vi "tearDown.vi"(8 "error in (no error)":errorcluster, 11 "LUnit test In":refnum<class "LUnit test 2.lvclass">) -> (0 "error out":errorcluster, 3 "LUnit test Out":refnum<class "LUnit test 2.lvclass">)   [LabVIEW 2020, in "LUnit test 2.lvclass"]
uses:
  LUnit test 2.lvclass
  <vilib>/Asteme/LUnit/Test Case.lvclass
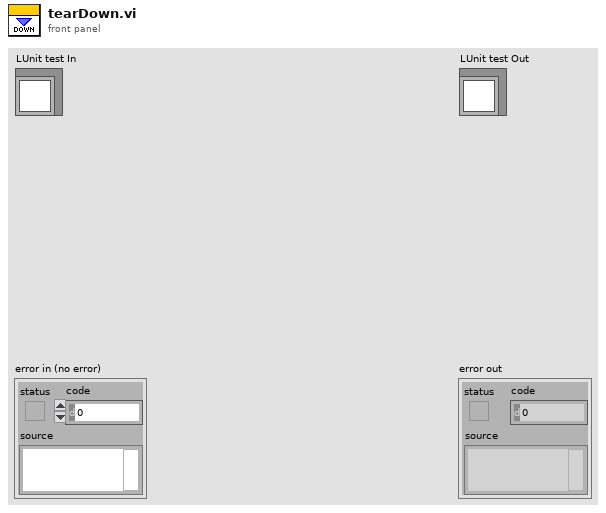
[diagram p1: front panel]
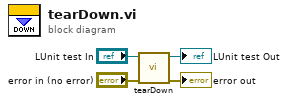
[diagram p0: block diagram]
diagram:
  n1 = call-parent "tearDown.vi"("error in (no error)"="error in (no error)", "LUnit Test Case In"="LUnit test In") -> ("error out"=→"error out":errorcluster, "LUnit Test Case Out"=→"LUnit test Out":refnum<class "LUnit test 2.lvclass">)  [unwired: 8 in]
